vi "Keith 7001 Chan Restrictions.vi"(0 "GPIB address":string="7", 1 "error in":T1, 2 "forbidden channel list":T2(array[cluster]) {"column" min=1; "channel/row" min=1; "slot/memory" min=1 max=2}, 3 "single channel mode":bool) -> (4 "error out":T1)   [LabVIEW 2019]
doc: "This VI sets up channel restrictions for the Keithley 7001 Switch System. The forbidden channel list specifies any channels which can not be closed. Any channels in the list which are closed before running will open once run. NOTE: resetting or turning off the device will not clear any forbidden channels in the unit's memory. To clear the memory, this VI must be run with an empty channel list.\n This VI also allows the operator to enable or disable the single channel mode. When enabled, only one channel can be closed at a time."
panel:
  # "enabled \ndisabled"
  # "memory location\nstandard channel"
  # "matrix card\nnon-matrix card"
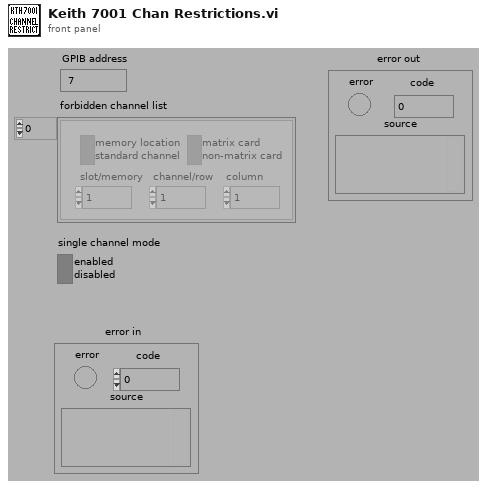
[diagram p1: front panel]
types:
  T1 = cluster{"error":bool, "code":i32, "source":string}
  T2 = cluster{"slot/memory":i16, "channel/row":i16, "column":i16, bool, bool}[]
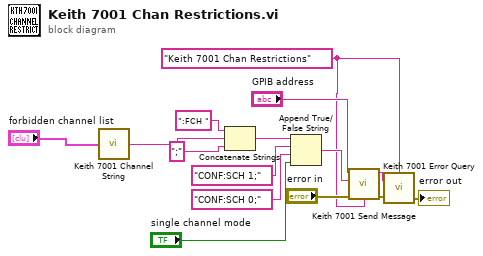
[diagram p0: block diagram]
diagram:
  w2 = "Keith 7001 Chan Restrictions"
  n1 = call "Keith 7001 Channel String.vi"("channel list"="forbidden channel list") -> (0:w8:string)
  n2 = Concatenate Strings(":FCH ", w8, ";") -> (w6:string)
  n3 = Append True/False String(1:"single channel mode", 2:"CONF:SCH 0;", 3:"CONF:SCH 1;", 4:w6) -> (0:w9:string)
  n4 = call "Keith 7001 Send Message.vi"("address string"="GPIB address", "write buffer"=w9, "source"=w2, "error in"="error in") -> ("address out"=w4:string, "error out"=w3:T1)  [unwired: 2 in, 2 out]
  n5 = call "Keith 7001 Error Query.vi"("GPIB address"=w4, "error in"=w3, "source"=w2) -> ("error out"=→"error out":T1)  [unwired: 2 out]
